vi "Check voltage and current.vi"(11 "VISA Refnum in":refnum<visa-resource-name>) -> ()   [LabVIEW 2020]
uses:
  Program Files/National Instruments/LabVIEW 2018/instr.lib/CAEN PSM/CAEN PSM.lvlib
panel:
  out "Voltage Channel 1":dbl
  out "Current Channel 1":dbl
  out "Current Channel 0":dbl
  out "Voltage Channel 0":dbl
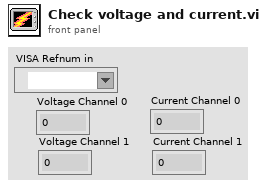
[diagram p1: front panel]
types:
  T1 = typedef "CAEN PSM.lvlib/BoardHandle.ctl" = cluster{"VISA resource name":refnum<visa-resource-name>, "Board address":u8, "NChannels":u8}
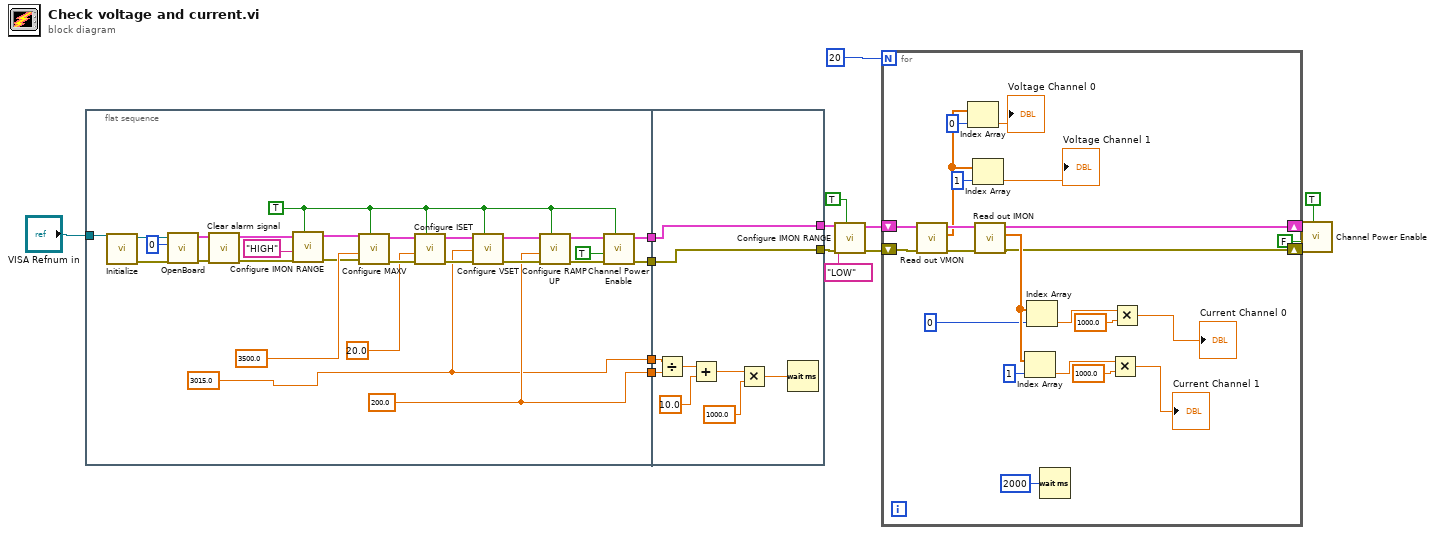
[diagram p0: block diagram]
diagram:
  n1 = flat-sequence {
    tunnel: [w17] -> w15
    tunnel: [w29] -> w14
    tunnel: [w28] -> w13
    tunnel: [w27] -> w12
    tunnel: "VISA Refnum in" -> [w26]
    tunnel: w15 -> [w47]
    tunnel: w14 -> [w46]
    tunnel: w13 -> [w45]
    tunnel: w12 -> [w44]
    tunnel: [w45] -> w6
    tunnel: [w44] -> _
    tunnel: [w44] -> w5
    frame #0 {
      w17 = 3015.0 ("x")
      w19 = TRUE ("All Channels (F)")
      w29 = 200.0 ("Voltage Ramp Up (V/s)")
      n2 = call "Initialize.vi"("VISA resource name"=w26) -> ("error out"=w38:errorcluster, "VISA resource name out"=w35:refnum<visa-resource-name>)  [unwired: 9 in]
      n3 = call "OpenBoard.vi"("error in (no error)"=w38, "Board Address"=u8 0, "VISA resource name"=w35) -> ("error out"=w39:errorcluster, "BoardHandle"=w34:T1)  [unwired: 7 in]
      n4 = call "Clear alarm signal.vi"("error in (no error)"=w39, "BoardHandle"=w34) -> ("error out"=w24:errorcluster, "BoardHandle out"=w23:T1)  [unwired: 8 in]
      n5 = call "Configure IMON RANGE.vi"("All Channels (F)"=w19, "error in (no error)"=w24, "IMon range (LOW)"="HIGH", "BoardHandle"=w23) -> ("error out"=w20:errorcluster, "BoardHandle out"=w21:T1)  [unwired: 6 in]
      n6 = call "Configure MAXV.vi"("All Channels (F)"=w19, "error in (no error)"=w20, "Voltage Max (0.0 V)"=3500.0 ("VMax (Volts)"), "BoardHandle"=w21) -> ("error out"=w40:errorcluster, "BoardHandle out"=w33:T1)  [unwired: 6 in]
      n7 = call "Configure ISET.vi"("All Channels (F)"=w19, "error in (no error)"=w40, "Current Limit (0.00 uA)"=20.0 ("Current Limit (uA)"), "BoardHandle"=w33) -> ("error out"=w41:errorcluster, "BoardHandle out"=w32:T1)  [unwired: 6 in]
      n8 = call "Configure VSET.vi"("All Channels (F)"=w19, "error in (no error)"=w41, "Voltage Level (0.0 V)"=w17, "BoardHandle"=w32) -> ("error out"=w42:errorcluster, "BoardHandle out"=w31:T1)  [unwired: 6 in]
      n9 = call "Configure RAMP UP.vi"("All Channels (F)"=w19, "error in (no error)"=w42, "Voltage ramp up (0 V/s)"=w29, "BoardHandle"=w31) -> ("error out"=w43:errorcluster, "BoardHandle out"=w30:T1)  [unwired: 6 in]
      n10 = call "Channel Power Enable.vi"("All Channels (F)"=w19, "error in (no error)"=w43, "Enable (OFF)"=TRUE ("Boolean"), "BoardHandle"=w30) -> ("error out"=w27:errorcluster, "BoardHandle out"=w28:T1)  [unwired: 6 in]
    }
    frame #1 {
      n11 = Divide(x=w47, y=w46) -> (x/y=w50:dbl)
      n12 = Add(x=w50, y=10.0) -> (x+y=w51:dbl)
      n13 = Multiply(x=w51, y=1000.0) -> (x*y=w52:dbl)
      n14 = Wait (ms)(milliseconds to wait=w52) -> ()  [unwired: 1 out]
    }
  }
  n15 = call "Configure IMON RANGE.vi"("All Channels (F)"=TRUE, "error in (no error)"=w5, "IMon range (LOW)"="LOW", "BoardHandle"=w6) -> ("error out"=w3:errorcluster, "BoardHandle out"=w4:T1)  [unwired: 6 in]
  n16 = for {
    N: 20 -> [_]
    shift-right: [w54] -> w10
    shift-left: w4 -> [w64]
    shift-right: [w55] -> w11
    shift-left: w3 -> [w63]
    n17 = call "Read out VMON.vi"("error in (no error)"=w63, "BoardHandle"=w64) -> ("error out"=w72:errorcluster, "VMon values (V)"=w56:dbl[], "BoardHandle out"=w71:T1)  [unwired: 7 in]
    n18 = Index Array(array=w56, index=0) -> (element=→"Voltage Channel 0":dbl)
    n19 = Index Array(array=w56, index=1) -> (element=→"Voltage Channel 1":dbl)
    n20 = call "Read out IMON.vi"("error in (no error)"=w72, "BoardHandle"=w71) -> ("error out"=w55:errorcluster, "IMon values (uA)"=w67:dbl[], "BoardHandle out"=w54:T1)  [unwired: 6 in, 1 out]
    n21 = Index Array(array=w67, index=1) -> (element=w69:dbl)
    n22 = Index Array(array=w67, index=0) -> (element=w73:dbl)
    n23 = Wait (ms)(milliseconds to wait=u32 2000) -> ()  [unwired: 1 out]
    n24 = Multiply(x=w69, y=1000.0) -> (x*y=→"Current Channel 1":dbl)
    n25 = Multiply(x=w73, y=1000.0) -> (x*y=→"Current Channel 0":dbl)
  }
  n26 = call "Channel Power Enable.vi"("All Channels (F)"=TRUE, "error in (no error)"=w11, "Enable (OFF)"=FALSE, "BoardHandle"=w10) -> ()  [unwired: 6 in, 2 out]
